vi "MVP02 GUID Lookup.vi"() -> ()   [LabVIEW 2016, in "MVP02 Custom Device.lvlib"]
doc: "Use this Global VI to access the GUIDs assigned to the page resources of the Custom Device."
uses:
  MVP02 Custom Device.lvlib
panel:
  in  "Custom Device":string="350c46f8-bd96-46af-8f1d-39f261e4859a"
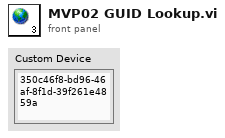
[diagram p1: front panel]
diagram:
